vi "TPNT_UpdateHdrs.vi"(8 "error in (no error)":errorcluster) -> (0 "error out":errorcluster)   [LabVIEW 2016]
uses:
  TPNT_CoreFunction.ctl
  DBSHAND/private/vis/DatabaseHand_Element_Get(bool).vi
  DBSHAND/private/vis/DatabaseHand_Element_Get(I32).vi
  DBSHAND/private/vis/DatabaseHand_Element_Set(3DArr).vi
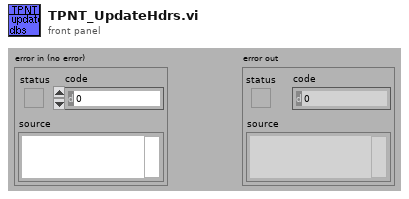
[diagram p1: front panel]
types:
  T1 = typedef "TPNT_CoreFunction.ctl" = enum16{"Reset", "Register", "Get Data", "Set Data", "Unregister", "Test", "Get Objects"}
  T2 = typedef "DatabaseHand_RefNum.ctl" = refnum<vi>
  T3 = enum16{"read from file", "get all", "clear all", "set file"}
  T4 = typedef "TPNT_Refnum.ctl" = refnum<vi>
  T5 = typedef "TPNT_DeviceTPs.ctl" = cluster{"device":string, "devupdate":dbl, "next_update":u32, "devinterface":string, "TPs":T6[], "Alarms":bool, "monitor":bool, "log sep":string}
  T6 = typedef "TPNT_TP.ctl" = cluster{"name":string, "type":string, "algor":string[], "update_rate":sgl, "Limits":T7, "Samples":T8, "next_update":u32, "Status":string, "monitor":bool, "error":bool, "Log":T9, "permissions":string, "ID":string}
  T7 = typedef "TPNT_Limits.ctl" = cluster{"Alarm Type":string, "Lower ":dbl, "Upper":dbl, "Nominal":dbl, "outrange":bool, "Check":bool, "latch":bool, "level":string}
  T8 = typedef "TPNT_Samples.ctl" = cluster{"samples":i32, "counter":i32, "Values":dbl[], "Current Value":string, "filter":string, "precision":u8}
  T9 = typedef "TPNT_Log.ctl" = cluster{"log":bool, "file":path, "type":string, "format":string, "updaterate":dbl, "nex_update":u32, "mode":string}
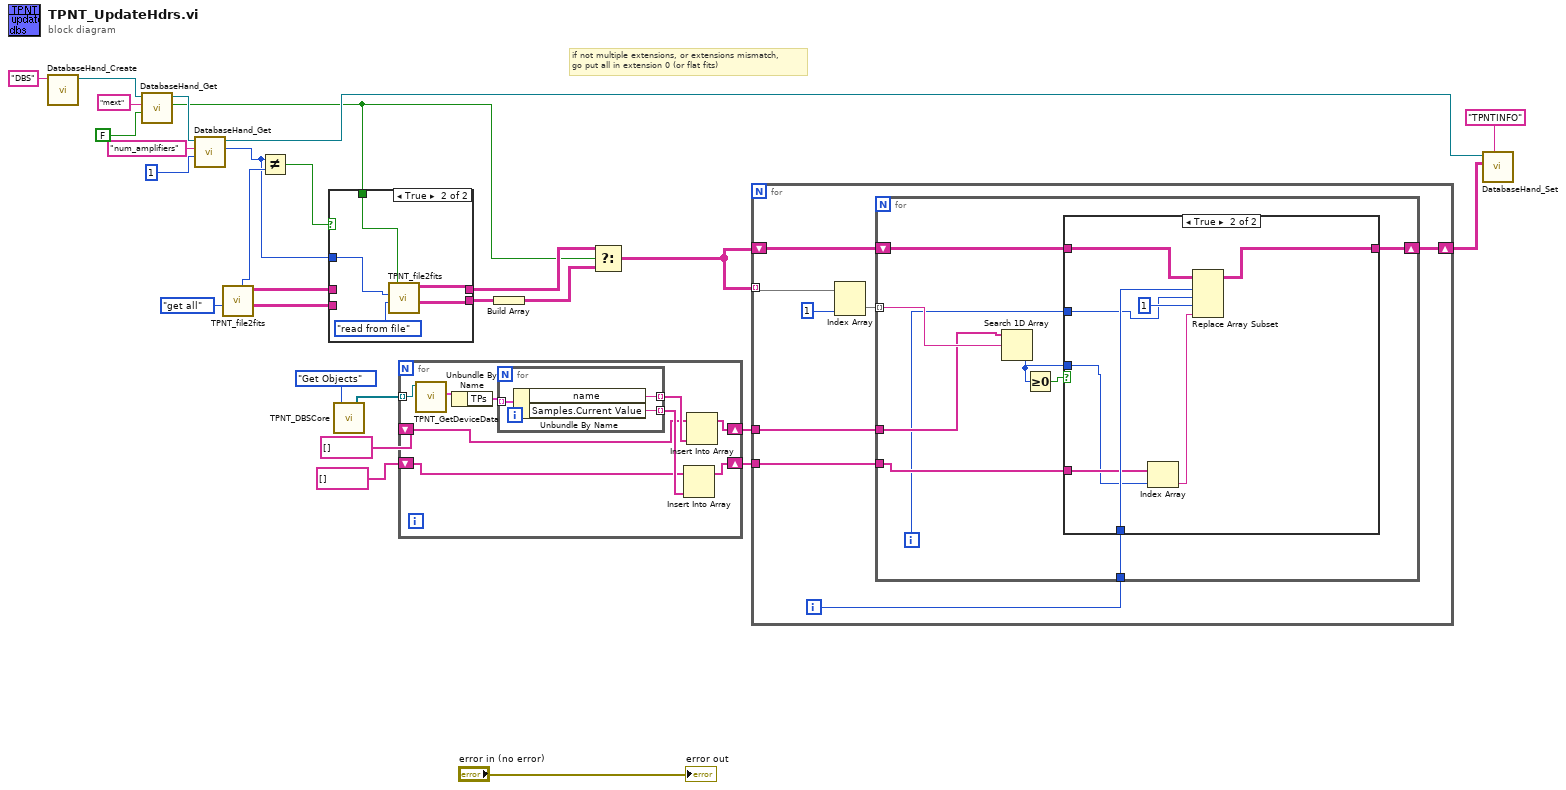
[diagram p0: block diagram]
diagram:
  # "if not multiple extensions, or extensions mismatch,\ngo put all in extension 0 (or flat fits)"
  n1 = call "DatabaseHand_Create.vi"("Name"="DBS") -> ("Database RefNum out"=w21:T2)  [unwired: 1 in, 9 out]
  n2 = call-poly "DatabaseHand_Get.vi"("default value"=FALSE, "name"="mext", "Database RefNum in"=w21) -> ("value"=w1:bool, "Database RefNum out"=w16:T2)  [unwired: 2 in, 5 out]
  n3 = call-poly "DatabaseHand_Get.vi"("default value"=1, "name"="num_amplifiers", "Database RefNum in"=w16) -> ("value"=w6:i32, "Database RefNum out"=w15:T2)  [unwired: 2 in, 5 out]
  n4 = call "TPNT_file2fits.vi"("action"=enum16{"read from file", "get all", "clear all"}."get all") -> ("flat keys"=w8:string[][], "Keywords"=w10:string[][][], "number of Extensions out"=w12:u16)  [unwired: 4 in, 4 out]
  n5 = Not Equal?(x=w6, y=w12) -> (x != y?=w11:bool)
  n6 = case shown="True" w11 {
    tunnel: w10 -> [w30 _]
    tunnel: [w30 w33] -> w9
    tunnel: w8 -> [w29 _]
    tunnel: [w29 w32] -> w7
    tunnel: w6 -> [_ w34]
    tunnel: w1 -> [_ w31]
    frame False {
    }
    frame True {
      n7 = call "TPNT_file2fits.vi"("mext"=w31, "action"=T3."read from file", "number of Extensions"=w34) -> ("flat keys"=w32:string[][], "Keywords"=w33:string[][][])  [unwired: 2 in, 5 out]
    }
  }
  n8 = call "TPNT_DBSCore.vi"("Function (Get Data)"=TPNT_CoreFunction."Get Objects") -> ("Objects"=w25:T4[])  [unwired: 4 in, 14 out]
  n9 = for {
    tunnel: w25 -> [w43] mode=indexing
    shift-right: [w41] -> w3
    shift-left: string[] [] -> [w37]
    shift-right: [w40] -> w2
    shift-left: string[] [] -> [w36]
    n10 = call "TPNT_GetDeviceData.vi"("Object Refnum In"=w43) -> ("Object Data Out"=w44:T5)  [unwired: 1 in, 9 out]
    n11 = Unbundle By Name(w44) -> ("TPs"=w42:T6[])
    n12 = for {
      tunnel: w42 -> [w47] mode=indexing
      tunnel: [w46] -> w39 mode=indexing
      tunnel: [w45] -> w38 mode=indexing
      n13 = Unbundle By Name(w47) -> ("name"=w46:string, "Samples.Current Value"=w45:string)
    }
    n14 = Insert Into Array(array=w36, new element=w38) -> (w40:string[])  [unwired: 1 in]
    n15 = Insert Into Array(array=w37, new element=w39) -> (w41:string[])  [unwired: 1 in]
  }
  n16 = Build Array(w7) -> (w17:string[][][])
  n17 = Select(t=w9, s=w1, f=w17) -> (s? t:f=w18:string[][][])
  n18 = for {
    tunnel: w18 -> [w55] mode=indexing
    shift-right: [w52] -> w22
    shift-left: w18 -> [w53]
    tunnel: w3 -> [w50]
    tunnel: w2 -> [w49]
    i -> [w51]
    n19 = Index Array(array=w55, index (col)=1 ("disabled index (col)")) -> (element=w48:string[])  [unwired: 1 in]
    n20 = for {
      tunnel: w48 -> [w59] mode=indexing
      shift-right: [w63] -> w52
      shift-left: w53 -> [w64]
      tunnel: w51 -> [w62]
      tunnel: w50 -> [w58]
      tunnel: w49 -> [w57]
      i -> [w56]
      n21 = Search 1D Array(1D array=w58, element=w59) -> (index of element=w61:i32)  [unwired: 1 out]
      n22 = Greater Or Equal To 0?(x=w61) -> (x >= 0?=w60:bool)
      n23 = case shown="True" w60 {
        tunnel: w64 -> [w65 w73]
        tunnel: [w65 w71] -> w63
        tunnel: w62 -> [_ w72]
        tunnel: w61 -> [_ w68]
        tunnel: w57 -> [_ w69]
        tunnel: w56 -> [_ w66]
        frame False {
        }
        frame True {
          n24 = Index Array(array=w69, index=w68) -> (element=w67:string)
          n25 = Replace Array Subset(array=w73, new element=w67, index (dim 0)=w72, index (dim 1)=w66, index (dim 2)=1 ("disabled index (col)")) -> (w71:string[][][])
        }
      }
    }
  }
  n26 = call-poly "DatabaseHand_Set.vi"("name"="TPNTINFO", "value"=w22, "Database RefNum in"=w15) -> ()  [unwired: 5 in, 4 out]
  "error out" <- "error in (no error)"
